vi "send_scanH_for_B_steps.vi"(0 "Instrument Ref In":refnum<k24>, 1 "Steps":dbl, 2 "Approach Mode":u16(ring) items=["Linear Approach", "No Overshoot Approach", "Oscillate Aproach"], 5 "Start Field":dbl, 7 "Rate":dbl, 9 "End Field":dbl, 11 "error in (no error)":errorcluster, 12 "Spacing Code":u16(ring) items=["Uniform spacing in field", "Uniform spacing in H^2"], 13 "PauseMode":u16(ring) items=["Persistent Mode", "Driven Mode"]) -> (4 "Instrument Ref Out":refnum<k24>, 15 "error out":errorcluster)   [LabVIEW 2019]
uses:
  C:/Software/CryoTUM/sub_vi-s/Equipment/PPMS/PPMSLabView/QDInstrument_LabVIEW/QDInstrument.dll
  Equipment/PPMS/PPMSLabView/QDInstrument_LabVIEW/QDInstrument.dll
panel:
  out "String":string
  out "ErrorReply":string
  out "PpmsReply":string
  out "SendPPMSCommand Error":i32
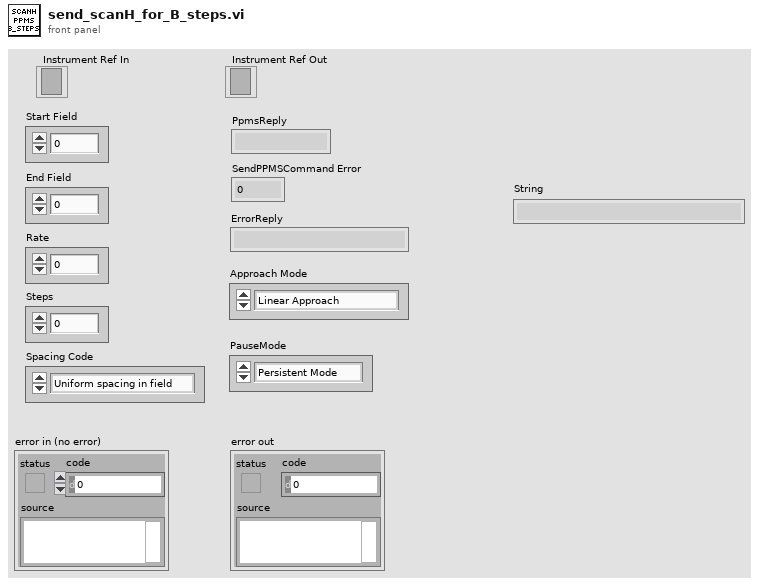
[diagram p1: front panel]
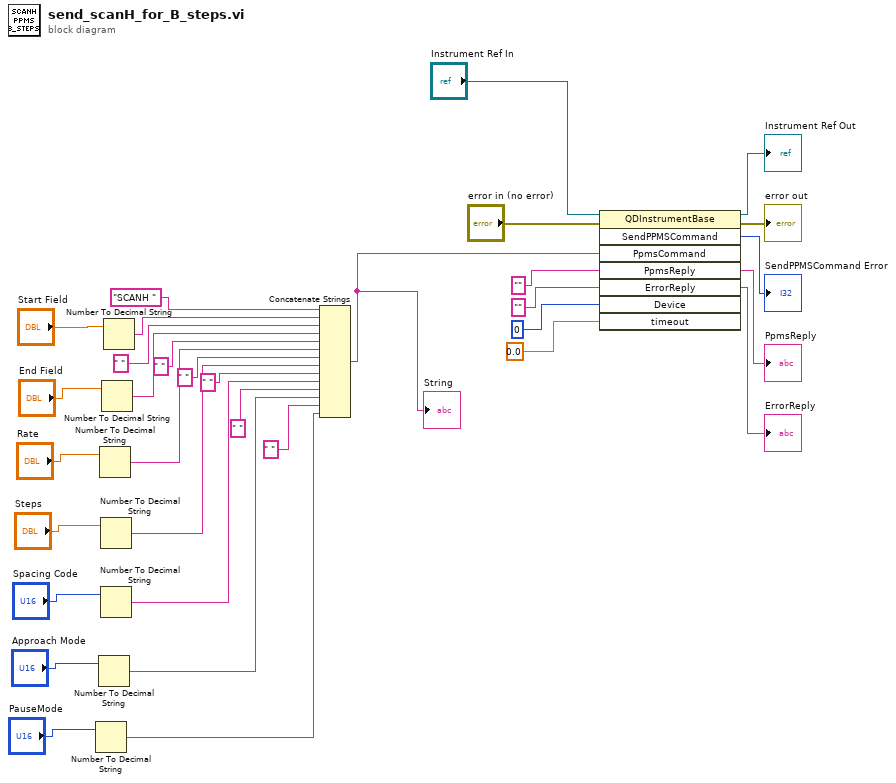
[diagram p0: block diagram]
diagram:
  n1 = Number To Decimal String(number="PauseMode") -> (decimal integer string=w4:string)  [unwired: 1 in]
  n2 = Number To Decimal String(number="Approach Mode") -> (decimal integer string=w6:string)  [unwired: 1 in]
  n3 = Number To Decimal String(number="Rate") -> (decimal integer string=w15:string)  [unwired: 1 in]
  n4 = Number To Decimal String(number="Steps") -> (decimal integer string=w12:string)  [unwired: 1 in]
  n5 = Number To Decimal String(number="Spacing Code") -> (decimal integer string=w9:string)  [unwired: 1 in]
  n6 = Number To Decimal String(number="End Field") -> (decimal integer string=w18:string)  [unwired: 1 in]
  n7 = Number To Decimal String(number="Start Field") -> (decimal integer string=w21:string)  [unwired: 1 in]
  n8 = Concatenate Strings("SCANH ", w21, " ", w18, " ", w15, " ", w12, " ", w9, " ", w6, " ", w4) -> (w2:string)
  "String" <- w2
  n9 = invoke class="QDInstrumentBase" method="SendPPMSCommand"(reference="Instrument Ref In", error in="error in (no error)", "PpmsCommand"=w2, "PpmsReply"="", "ErrorReply"="", "Device"=0, "timeout"=0.0 ("Result")) -> (reference out=→"Instrument Ref Out":refnum<k24>, error out=→"error out":errorcluster, "SendPPMSCommand"=→"SendPPMSCommand Error":i32, "PpmsReply"=→"PpmsReply":string, "ErrorReply"=→"ErrorReply":string)  [unwired: 1 in, 3 out]
